vi "SRS_QCM_SubVI  11-08-2017.vi"(0 "VISA Refnum in":refnum<visa-resource-name>, 1 "first iteration?":bool, 5 "Frequency  in":dbl, 7 "SRS on?":bool, 11 "error in (no error)":errorcluster) -> (3 "Frequency out 2":dbl, 4 "freq, mass, MR":T1, 6 "Frequency out":dbl format="%#_8g", 8 "address out":T3, 10 "M":string, 13 "MR":string, 14 "F":string, 15 "M,F,MR output cluster":T2)   [LabVIEW 2014]
panel:
  out "error out":errorcluster
  in  "VISA in":refnum<visa-resource-name>="GPIB0::3::INSTR"
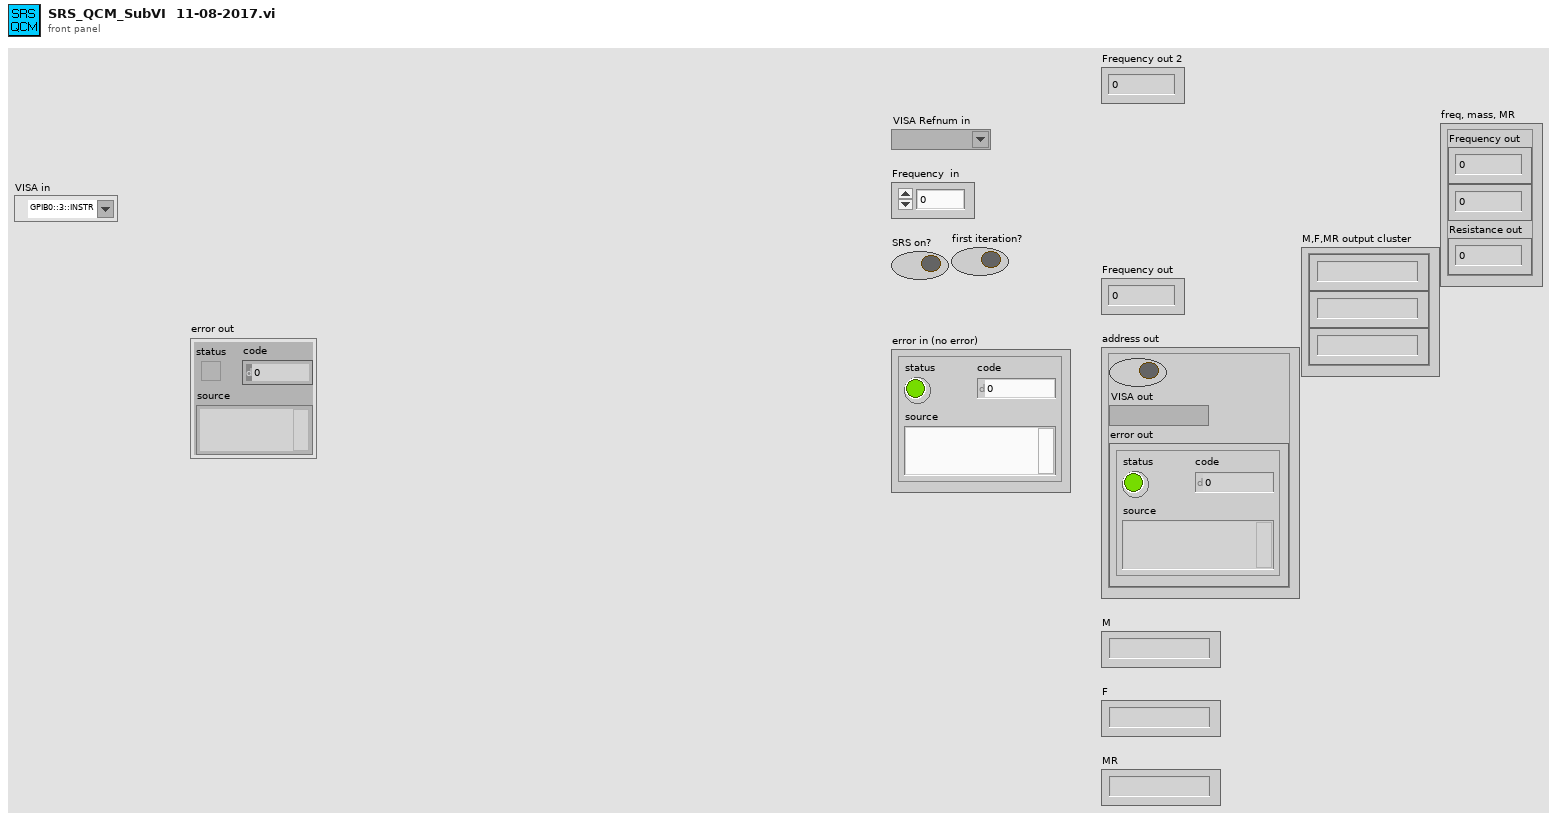
[diagram p1: front panel]
types:
  T1 = cluster{"Frequency out":dbl, "Numeric Control":dbl, "Resistance out":dbl}
  T2 = cluster{"String":string, "String":string, "String":string}
  T3 = cluster{"Boolean":bool, "VISA out":refnum<visa-resource-name>, "error out":errorcluster}
  T4 = cluster{"SRS on?":bool, "VISA out":refnum<visa-resource-name>, "error out":errorcluster}
  T5 = cluster{dbl, "Frequency out":dbl, "Resistance out":dbl}
  T6 = cluster{"Frequency out":dbl, dbl, "Resistance out":dbl}
  T7 = cluster{string, "Frequency out":string, "Resistance out":string}
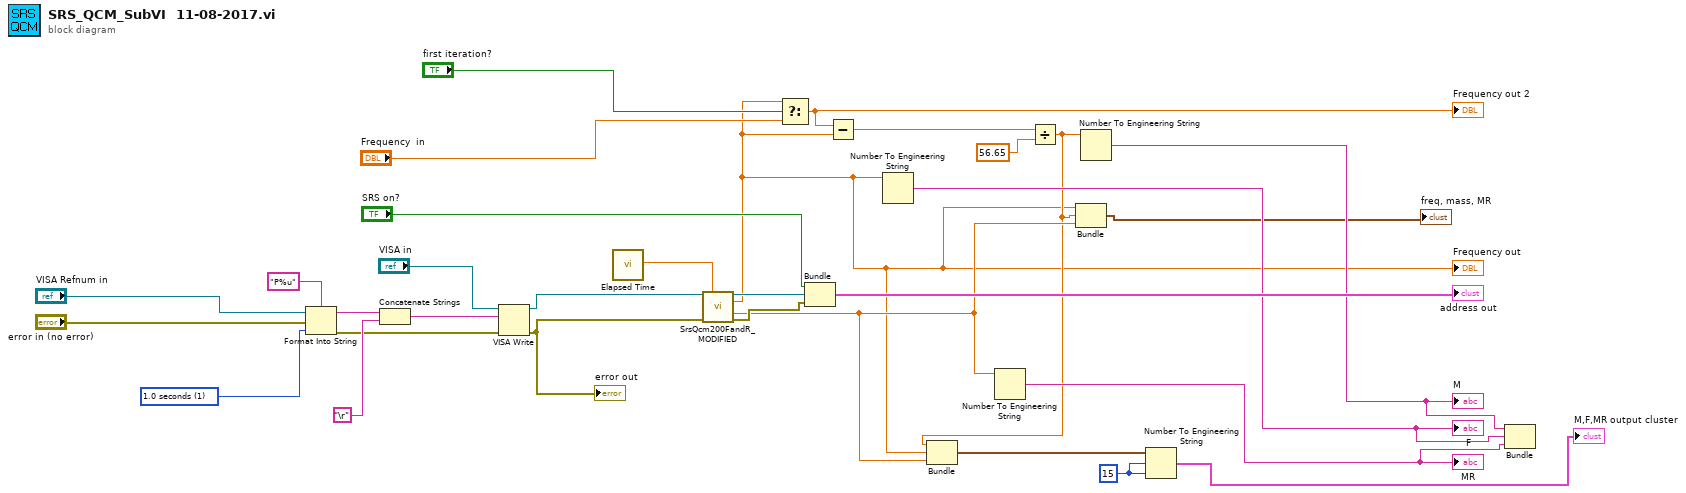
[diagram p0: block diagram]
diagram:
  w5 = u16 1 items=["0.1 seconds", "1.0 seconds", "10.0 seconds"] ("Gate time 2")
  w15 = i16 15 ("width (-)")
  n1 = Format Into String(format string="P%u", initial string="VISA Refnum in", error in="error in (no error)", w5) -> (resulting string=w6:string, error out=w7:errorcluster)
  n2 = Concatenate Strings(w6, "\r") -> (w9:string)
  n3 = VISA Write(VISA resource name="VISA in", write buffer=w9, error in (no error)=w7) -> (VISA resource name out=w1:refnum<visa-resource-name>, error out=w2:errorcluster)  [unwired: 1 out]
  "error out" <- w2
  n4 = call "Elapsed Time"() -> ("Elapsed Time (s)"=w25:dbl)  [unwired: 12 in, 7 out]
  n5 = call "SrsQcm200FandR_MODIFIED.vi"("VISA in"=w1, "Reference time in"=w25, "error in (no error)"=w2) -> ("VISA out"=w27:refnum<visa-resource-name>, "Frequency out"=w13:dbl, "Resistance out"=w18:dbl, "error out"=w26:errorcluster)  [unwired: 6 in, 3 out]
  "Frequency out" <- w13
  n6 = Select(t=w13, s="first iteration?", f="Frequency  in") -> (s? t:f=w31:dbl)
  "Frequency out 2" <- w31
  n7 = Bundle("SRS on?"="SRS on?", "VISA out"=w27, "error out"=w26) -> (→"address out":T4)  [unwired: 1 in]
  n8 = Subtract(x=w31, y=w13) -> (x-y=w29:dbl)
  n9 = Number To Engineering String(4:w13) -> (0:w19:string)  [unwired: 3 in]
  "F" <- w19
  n10 = Number To Engineering String(4:w18) -> (0:w20:string)  [unwired: 3 in]
  "MR" <- w20
  n11 = Divide(x=w29, y=56.65) -> (x/y=w14:dbl)
  n12 = Bundle(w14, "Frequency out"=w13, "Resistance out"=w18) -> (w17:T5)  [unwired: 1 in]
  n13 = Bundle("Frequency out"=w13, w14, "Resistance out"=w18) -> (→"freq, mass, MR":T6)  [unwired: 1 in]
  n14 = Number To Engineering String(4:w14) -> (0:w21:string)  [unwired: 3 in]
  "M" <- w21
  n15 = Number To Engineering String(2:w15, 3:w15, 4:w17) -> (0:→"M,F,MR output cluster":T7)  [unwired: 1 in]
  n16 = Bundle(w21, w19, w20) -> ()  [unwired: 1 in, 1 out]
